vi "WILT Station Save.vi"(6 "Test Station State":string, 7 "Dryer 14":T1 {"Night Cycle Count" format="%04d"; "Day Cycle Count" format="%04d"}, 8 "error in (no error)":errorcluster, 9 "First Time Through?":bool, 10 "File Locations A":T5, 11 "Byte Stream File in":refnum<file>) -> (0 "error out":errorcluster, 1 "First Time Through Out":bool, 2 "File Path Output New out":T5, 3 "Byte Stream File out":refnum<file>, 5 "New File?":bool)   [LabVIEW 2016]
uses:
  Utility/Save File/File Setup (Public)/Type Definition/Save File DOE File Path Control.ctl
  Utility/Save File/File Setup (Public)/Type Definition/Save File DOE Data Save Filepaths.ctl
  Type Definitions/WILT Dryer.ctl
  Type Definitions/WILT Dryer Details.ctl
  Type Definitions/WILT Agilent Channel Definition.ctl
  Type Definitions/WILT DAQ Data.ctl
  Utility/Save File/File Setup (Public)/Type Definition/Save File DOE LabView Program.ctl
  Utility/Save File/Save File.lvlib
  Utility/Save File/File Setup.lvlib
panel:
  # "Day"
  # "Night"
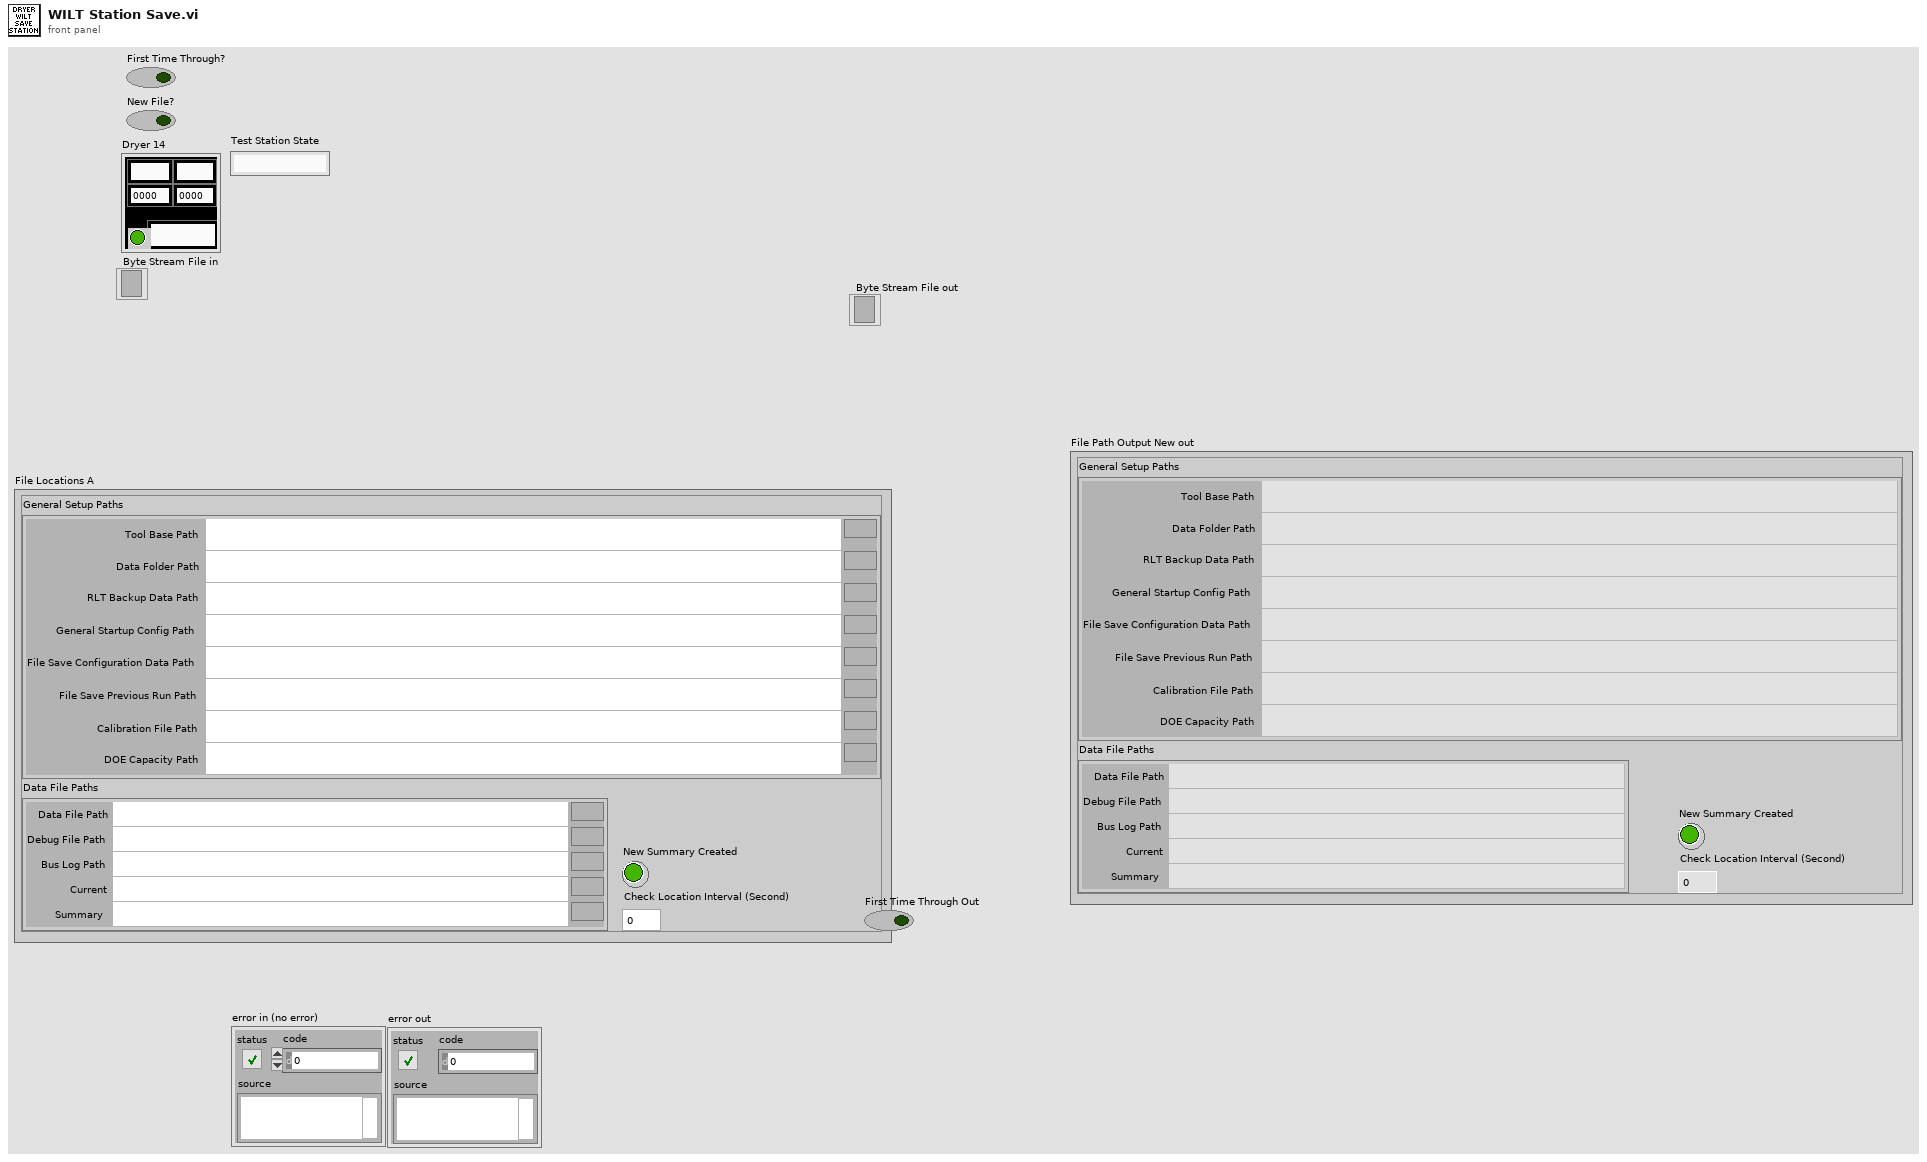
[diagram p1: front panel]
types:
  T1 = typedef "WILT Dryer.ctl" = cluster{"Lab ID":string, "Day Cycle Count":i32, "Station Label":string, "Dryer Details":T2, "Status Color":u32, "Invisible Button":bool, "Night Cycle Count":i32, "Station Index":i32, "Cycle Index":string, "Audit Alert":bool, "Agilent Channel Definition":T3, "DAQ Data":T4}
  T2 = typedef "WILT Dryer Details.ctl" = cluster{"Station":string, "Lab ID":string, "TR Number":string}
  T3 = typedef "WILT Agilent Channel Definition.ctl" = cluster{"Channel":string, "Station":string, "Label":string, "Agilent Station":string, "Data":dbl}
  T4 = typedef "WILT DAQ Data.ctl" = cluster{"L1 Current":dbl, "L2 Current":dbl, "Temperature  Deg F (TC)":dbl, "Volts":dbl, "Volts (208)":dbl, "SW (208)":dbl}
  T5 = typedef "File Setup.lvlib/Save File DOE File Path Control.ctl" = cluster{"General Setup Paths":cluster{"Calibration File Path":path, "DOE Capacity Path":path, "Data Folder Path":path, "RLT Backup Data Path":path, "Tool Base Path":path, "General Startup Config Path":path, "File Save Previous Run Path":path, "File Save Configuration Data Path":path}, "Data File Paths":T6, "New Summary Created":bool, "Check Location Interval (Second)":i32}
  T6 = typedef "File Setup.lvlib/Save File DOE Data Save Filepaths.ctl" = cluster{"Data File Path":path, "Debug File Path":path, "Bus Log Path":path, "Current":path, "Summary":path}
  T7 = typedef "File Setup.lvlib/Save File DOE LabView Program.ctl" = enum16{"No Name Found", "DOE Stand", "Dishwasher Kitchen", "Portable Stand", "HEWH", "Dryer", "Dryer WILT", "HCC", "PRAT", "HEWH RLT", "Refrigeration"}
  T8 = typedef "Save File.lvlib/Save File Washer.ctl" = cluster{"Appliance Details":T9, "Display Data (RLT)":T15}
  T9 = typedef "File Setup.lvlib/Save File DISH Dishwasher Details.ctl" = cluster{"FileVersionInfo":T10, "Dishwasher Info":cluster{"Open Cup Weight (gm):":dbl, "Auto Cup Weight (gm):":dbl, "Detergent-Dish:":string, "Inlet Temperature-Dish:":string, "Cycle Mode-Dish:":string, "Unit Control-Dish:":string, "Manufacturer-Dish:":string}, "Washer Info":cluster{"Hot Water Temperature (Fahrenheit):":string, "Cold Water Temperature (Fahrenheit):":string, "Capacity (cu.ft):":dbl, "Initial Cloth Weight:":dbl, "Cloth Lot:":i32, "Model Family:":string, "Program Name:":string, "Cycle Selection:":string, "Wash Temperature:":string, "Rinse Temperature:":string, "Load Size:":string}, "File Name Output Array":string[][], "Calibration Output Array":string[][], "Appliance Common":T11, "Water Heater":cluster{"Heating Mode:":string}, "Dryer":cluster{"Heat Setting:":T12, "Washer Water Temperature (60 ± 5°F):":u16, "Water Hardness (PPM):":u16, "Dryness Setting:":T12, "Dryer Type:":string, "Exhaust:":string, "Drying Cycle:":string, "Load Type:":string, "Nominal Load Weight":string, "Dryer Initial IMC Data":T13}}
  T10 = typedef "FileVersionInformation.ctl" = cluster{"FileVersion":string, "ProductName":string, "InternalName":string, "CompanyName":string, "LegalCopyright":string, "FileDescription":string}
  T11 = typedef "DOE Appliance Common.ctl" = cluster{"Engineer:":string, "Model Number:":string, "Serial Number:":string, "Comments:":string, "Station ID:":string, "Technician:":string, "TR Number:":string, "Lab ID:":string, "Voltage:":string, "Water Pressure (PSI):":string, "Test Date:":string, "Computer Name:":string, "IP Address:":string, "Ambient RH:":string, "Frequency:":string, "Build:":string, "Filename:":string, "Test Type:":string, "Load Run #:":i32, "Ambient Temperature (F):":string, "File Path:":path, "Cycles Per Year":u32}
  T12 = typedef "Custom Pallet String.ctl" = string
  T13 = typedef "DPT IMC Data.ctl" = cluster{"Measured IMC (lbs)":dbl, "Actual Initial RMC (%)":dbl, "RMC (Desired %)":dbl, "Bone Dry Wt(lbs)":dbl, "Tolerance(%)":dbl, "Actual Final RMC (%)":dbl, "CEF (lbf/kWh)":dbl, "Minimum Weight (lbf)":dbl, "Average Weight (lbf)":dbl, "Maximum Weight (lbf)":dbl, "Measured IMC In Range?":bool, "Moisture Reduction Factor":dbl, "Field Use Factor":dbl, "Empty Dryer Cold Weigth":dbl, "Energy Standard":T14, "Weight Cloth (lbs)":dbl, "Relative Moisture Content (%)":dbl, "Relative Moisture Content - Avg (%)":dbl}
  T14 = typedef "DOE Dryer Standard.ctl" = enum16{"D2-Automatic Dryer", "D2-Timer Dryer", "D1-Automatic Dryer", "D1-Timer Dryer", "Other"}
  T15 = typedef "Save File Appliance Display.ctl" = cluster{"Status Color":u32, "Serial Number Display":string, "Cycle Count Display":i32, "Station Label Display":string, "Current Run Start Time Display":dbl, "Board ID Display":string, "RPM Display":u32, "Current Display":dbl, "Current Path Display":path, "Saving Display":bool, "Unit Type Display":T16, "Total Time On Display":dbl, "UI Button":bool}
  T16 = typedef "Save File.lvlib/Save File Unit Type.ctl" = enum32{"", "Viper", "Hawk", "2015"}
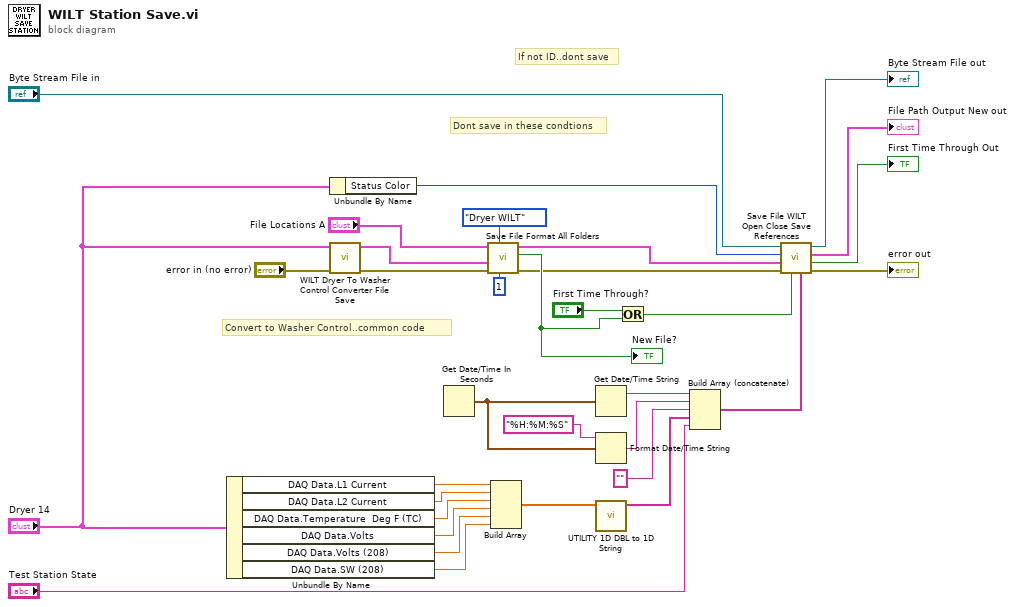
[diagram p0: block diagram]
diagram:
  # "Dont save in these condtions"
  # "If not ID..dont save"
  # "Convert to Washer Control..common code"
  n1 = Unbundle By Name("Dryer 14") -> ("DAQ Data.L1 Current"=w10:dbl, "DAQ Data.L2 Current"=w11:dbl, "DAQ Data.Temperature  Deg F (TC)"=w12:dbl, "DAQ Data.Volts"=w13:dbl, "DAQ Data.Volts (208)"=w14:dbl, "DAQ Data.SW (208)"=w15:dbl)
  n2 = Unbundle By Name("Dryer 14") -> ("Status Color"=w3:u32)
  n3 = call "WILT Dryer To Washer Control Converter File Save.vi"("Error In"="error in (no error)", "Dryer 14"="Dryer 14") -> ("Error Out"=w6:errorcluster, "Initialize.Washer In"=w9:T8)  [unwired: 8 in]
  n4 = Get Date/Time In Seconds() -> (seconds since 1Jan1904=w22:timestamp)
  n5 = call "Save File Format All Folders.vi"("Number of Cycles/ File"=1, "LV Program"=Save_File_DOE_LabView_Program."Dryer WILT", "error in (no error)"=w6, "Initialize.Washer In"=w9, "File Locations In"="File Locations A") -> ("error out"=w5:errorcluster, "New File?"=w26:bool, "File Locations Out"=w28:T5)  [unwired: 4 in]
  "New File?" <- w26
  n6 = Build Array(w10, w11, w12, w13, w14, w15) -> (w19:dbl[])
  n7 = Get Date/Time String(seconds (now)=w22) -> (date string=w23:string)  [unwired: 2 in, 1 out]
  n8 = Format Date/Time String(time format string (%c)="%H:%M:%S", seconds (now)=w22) -> (date/time string=w24:string)  [unwired: 1 in]
  n9 = call "UTILITY 1D DBL to 1D String.vi"("1D DBL"=w19) -> ("1D String"=w20:string[])  [unwired: 10 in]
  n10 = Or(x="First Time Through?", y=w26) -> (x .or. y?=w16:bool)
  n11 = Build Array (concatenate)(w23, w24, "" ("element"), w20, "Test Station State") -> (w25:string[])
  n12 = call "Save File WILT Open Close Save References.vi"("Save Data"=w25, "New File?"=w16, "error in (no error)"=w5, "File Path Output New in"=w28, "Status Color"=w3, "Byte Stream File in"="Byte Stream File in") -> ("error out"=→"error out":errorcluster, "First Time Through Out"=→"First Time Through Out":bool, "File Path Output New out"=→"File Path Output New out":T5, "Byte Stream File out"=→"Byte Stream File out":refnum<file>)  [unwired: 2 in]
